vi "Add Extra Page to System Explorer.vi"(6 "SE Path Cluster In":T3, 7 "Pages Properties":T1[](array[typedef]), 8 "error in":errorcluster, 9 "DLL Path":path) -> (0 "error out":errorcluster, 4 "SE Path Cluster In":T3, 5 "Pages Properties Out":T1[](array[typedef]))   [LabVIEW 2026, in "NIVS_CDEW_MetaDataObj.lvclass"]
uses:
  NIVS_CDEW_MetaDataObj.lvclass
  Types/Page Properties.ctl
  NIVS_CDEW_MetaDataObj.lvclass/NIVS_CDEW_MetaDataObj.ctl
  Types/Page Types.ctl
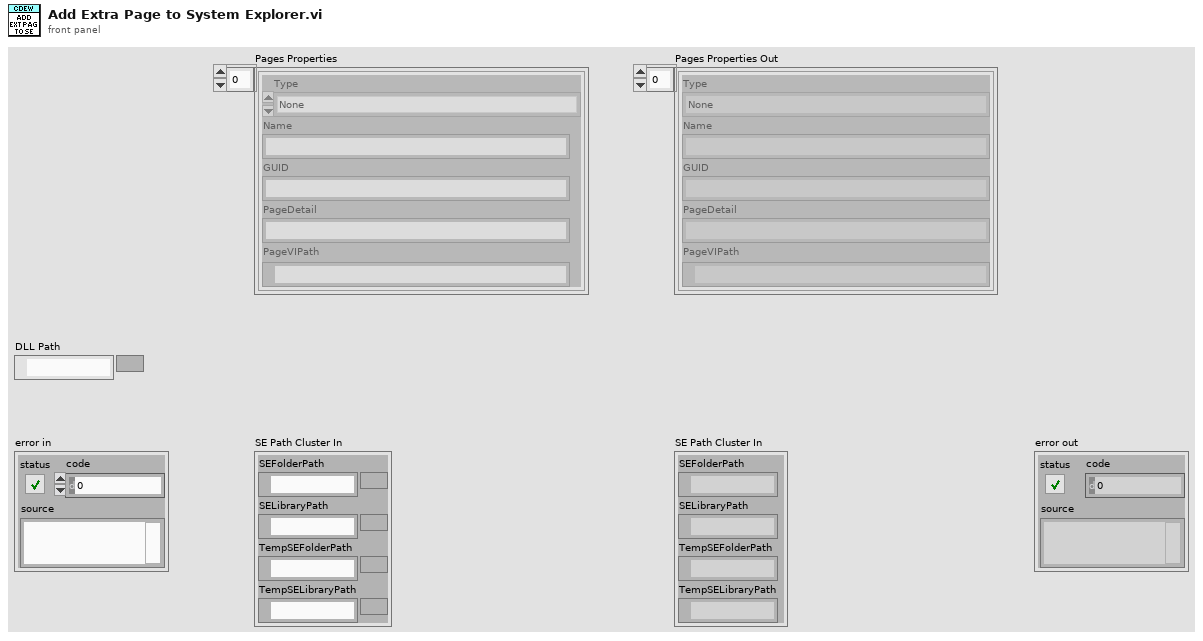
[diagram p1: front panel]
types:
  T1 = typedef "NIVS_CDEW_MetaDataObj.lvclass/Page Properties.ctl" = cluster{"Type":T2, "Name":string, "GUID":string, "PageDetail":string, "PageVIPath":path}
  T2 = typedef "NIVS_CDEW_MetaDataObj.lvclass/Page Types.ctl" = enum16{"None", "CustomDevice", "Channel", "Waveform", "Section", "DynamicChannel", "DynamicWaveform", "DynamicSection"}
  T3 = cluster{"SEFolderPath":path, "SELibraryPath":path, "TempSEFolderPath":path, "TempSELibraryPath":path}
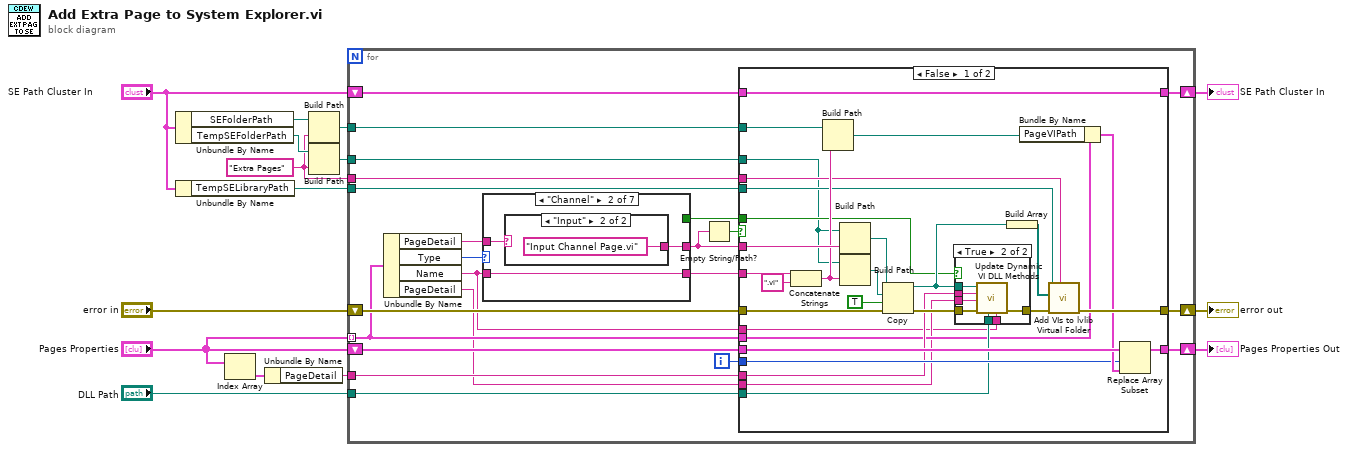
[diagram p0: block diagram]
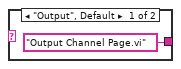
[diagram p5: hidden frame]
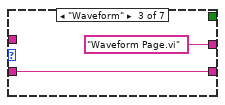
[diagram p6: hidden frame]
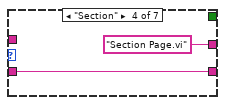
[diagram p7: hidden frame]
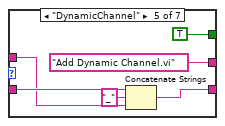
[diagram p8: hidden frame]
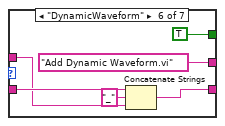
[diagram p9: hidden frame]
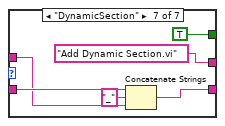
[diagram p10: hidden frame]
diagram:
  w3 = "Extra Pages" ("Virtual Folder Name")
  n1 = Unbundle By Name("SE Path Cluster In") -> ("SEFolderPath"=w7:path, "TempSEFolderPath"=w5:path)
  n2 = Unbundle By Name("SE Path Cluster In") -> ("TempSELibraryPath"=w1:path)
  n3 = Index Array(array="Pages Properties") -> (element=w9:T1)  [unwired: 1 in]
  n4 = Unbundle By Name(w9) -> ("PageDetail"=w8:string)
  n5 = Build Path(base path=w7, name or relative path=w3) -> (appended path=w6:path)
  n6 = Build Path(base path=w5, name or relative path=w3) -> (appended path=w4:path)
  n7 = for {
    tunnel: "Pages Properties" -> [w30] mode=indexing
    shift-right: [w36] -> w14
    shift-left: "error in" -> [w37]
    shift-right: [w31] -> w15
    shift-left: "SE Path Cluster In" -> [w35]
    shift-right: [w27] -> w12
    shift-left: "Pages Properties" -> [w29]
    tunnel: "DLL Path" -> [w26]
    tunnel: w8 -> [w25]
    tunnel: w6 -> [w19]
    tunnel: w4 -> [w18]
    tunnel: w3 -> [w17]
    tunnel: w1 -> [w16]
    i -> [w28]
    n8 = Unbundle By Name(w30) -> ("PageDetail"=w23:string, "Type"=w34:T2, "Name"=w20:string, "PageDetail"=w22:string)
    n9 = case shown="\"Channel\"" w34 {
      tunnel: [_ w78 "Waveform Page.vi" ("string") "Section Page.vi" ("string") "Add Dynamic Channel.vi" ("string") "Add Dynamic Waveform.vi" ("string") "Add Dynamic Section.vi" ("string")] -> w33
      tunnel: w23 -> [_ w79 _ _ w87 w93 w99]
      tunnel: [_ _ _ _ TRUE TRUE TRUE] -> w24
      tunnel: [_ w80 w83 w85 w88 w94 w100] -> w21
      tunnel: w20 -> [_ w80 w83 w85 w89 w95 w101]
      frame "None", "CustomDevice" {
      }
      frame "Channel" {
        n10 = case shown="\"Input\"" w79 {
          tunnel: ["Output Channel Page.vi" ("string") "Input Channel Page.vi" ("string")] -> w78
          frame "Output", Default {
          }
          frame "Input" {
          }
        }
      }
      frame "Waveform" {
      }
      frame "Section" {
      }
      frame "DynamicChannel" {
        n11 = Concatenate Strings(w89, "_" ("string"), w87) -> (w88:string)
      }
      frame "DynamicWaveform" {
        n12 = Concatenate Strings(w95, "_" ("string"), w93) -> (w94:string)
      }
      frame "DynamicSection" {
        n13 = Concatenate Strings(w101, "_" ("string"), w99) -> (w100:string)
      }
    }
    n14 = Empty String/Path?(string/path=w33) -> (empty?=w32:bool)
    n15 = case shown="False" w32 {
      tunnel: w21 -> [w49 _]
      tunnel: w37 -> [w66 w76]
      tunnel: [w65 w76] -> w36
      tunnel: w35 -> [w58 w77]
      tunnel: w33 -> [w59 _]
      tunnel: [w58 w77] -> w31
      tunnel: w30 -> [w44 _]
      tunnel: w29 -> [w57 w75]
      tunnel: w28 -> [w55 _]
      tunnel: [w54 w75] -> w27
      tunnel: w19 -> [w41 _]
      tunnel: w18 -> [w38 _]
      tunnel: w26 -> [w50 _]
      tunnel: w25 -> [w48 _]
      tunnel: w24 -> [w45 _]
      tunnel: w22 -> [w43 _]
      tunnel: w20 -> [w42 _]
      tunnel: w17 -> [w40 _]
      tunnel: w16 -> [w39 _]
      frame False {
        n16 = Concatenate Strings(w49, ".vi" ("string")) -> (w53:string)
        n17 = Build Path(base path=w41, name or relative path=w53) -> (appended path=w52:path)
        n18 = Build Path(base path=w38, name or relative path=w59) -> (appended path=w60:path)
        n19 = Build Path(base path=w38, name or relative path=w53) -> (appended path=w63:path)
        n20 = Copy(8:w66, 9:TRUE ("overwrite (F)"), 10:w63, 11:w60) -> (0:w51:errorcluster, 3:w47:path)  [unwired: 1 in, 1 out]
        n21 = case shown="True" w45 {
          tunnel: w51 -> [w67 w74]
          tunnel: w50 -> [_ w73]
          tunnel: w42 -> [_ w72]
          tunnel: w48 -> [_ w71]
          tunnel: w43 -> [_ w70]
          tunnel: w47 -> [_ w69]
          tunnel: [w67 w68] -> w46
          frame False {
          }
          frame True {
            n22 = call "Update Dynamic VI DLL Methods.vi"("MethodName"=w72, "DLL Path"=w73, "error in"=w74, "Custom Device Name"=w70, "NameSpace"=w71, "VI path"=w69) -> ("error out"=w68:errorcluster)  [unwired: 5 in]
          }
        }
        n23 = Build Array(w47) -> (w61:path[])
        n24 = Bundle By Name(cluster=w44, "PageVIPath"=w52) -> (w56:T1)
        n25 = call "Add VIs to lvlib Virtual Folder.vi"("Virtual Folder Name"=w40, "error in"=w46, "VIs to add"=w61, "lvlib Path"=w39) -> ("error out"=w65:errorcluster)  [unwired: 7 in]
        n26 = Replace Array Subset(array=w57, new element=w56, index=w55) -> (w54:T1[])
      }
      frame True {
      }
    }
  }
  "SE Path Cluster In" <- w15
  "error out" <- w14
  "Pages Properties Out" <- w12
